vi "controlRealtimeInputMove.vi"(7 "Set":bool, 8 "error in":errorcluster, 9 "move in":bool=TRUE, 10 "axis in":u8, 11 "connection ID":refnum<k5>) -> (0 "error out":errorcluster, 1 "move out":bool=TRUE, 2 "axis out":u8, 3 "connection ID":refnum<k5>)   [LabVIEW 2016]
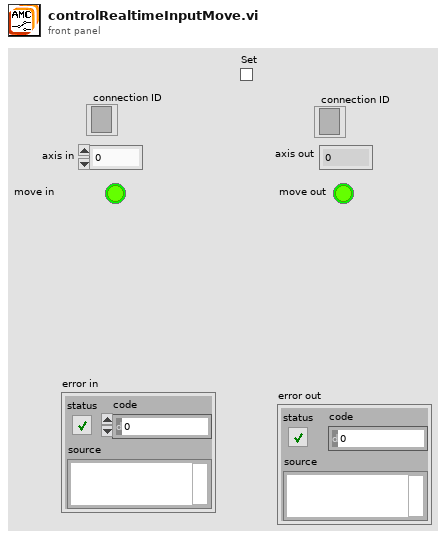
[diagram p1: front panel]
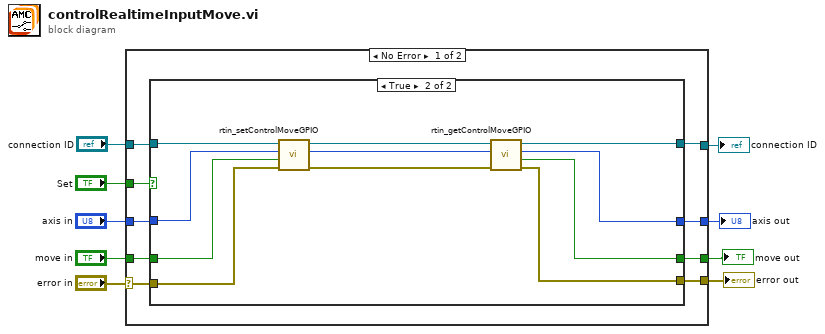
[diagram p0: block diagram]
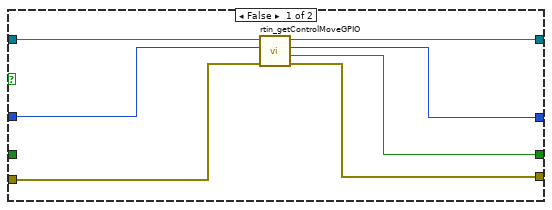
[diagram p2: hidden frame]
diagram:
  n1 = case shown="No Error" "error in" {
    selector: "error in" -> [w10 w40]
    tunnel: "axis in" -> [w16 w38]
    tunnel: [w11 w40] -> w8
    tunnel: [w13 w38] -> w7
    tunnel: "Set" -> [w17 _]
    tunnel: "move in" -> [w15 w39]
    tunnel: [w14 w37] -> w4
    tunnel: "connection ID" -> [w18 w37]
    tunnel: [w12 w39] -> w2
    frame No Error {
      n2 = case shown="True" w17 {
        tunnel: [w24 w28] -> w14
        tunnel: w18 -> [w25 w36]
        tunnel: w16 -> [w21 w34]
        tunnel: [w20 w29] -> w13
        tunnel: [w22 w31] -> w11
        tunnel: [w19 w30] -> w12
        tunnel: w15 -> [_ w33]
        tunnel: w10 -> [w23 w35]
        frame False {
          n3 = call "rtin_getControlMoveGPIO.vi"("error in"=w23, "axis"=w21, "connection ID"=w25) -> ("error out"=w22:errorcluster, "enable"=w19:bool, "axis_out"=w20:i32, "connection ID"=w24:refnum<k5>)  [unwired: 5 in]
        }
        frame True {
          n4 = call "rtin_setControlMoveGPIO.vi"("error in"=w35, "enable"=w33, "axis"=w34, "connection ID"=w36) -> ("error out"=w32:errorcluster, "axis_out"=w26:i32, "connection ID"=w27:refnum<k5>)  [unwired: 5 in]
          n5 = call "rtin_getControlMoveGPIO.vi"("error in"=w32, "axis"=w26, "connection ID"=w27) -> ("error out"=w31:errorcluster, "enable"=w30:bool, "axis_out"=w29:i32, "connection ID"=w28:refnum<k5>)  [unwired: 5 in]
        }
      }
    }
    frame Error {
    }
  }
  "error out" <- w8
  "axis out" <- w7
  "move out" <- w2
  "connection ID" <- w4
